vi "Launch.vi"(8 "error in (no error)":errorcluster, 10 "Mediator":refnum<class "IMediator.lvclass">, 11 "IMediatorBusMonitor (Type)":refnum<class "IMediatorBusMonitor.lvclass">) -> (0 "error out":errorcluster, 1 "Bus Monitor Enqueuer":refnum<class "Message Enqueuer.lvclass">, 2 "Mediator Out":refnum<class "IMediator.lvclass">, 3 "Notification Msg Type":refnum<class "Notification Msg.lvclass">)   [LabVIEW 2017, in "IMediator.lvlib" / "IMediatorBusMonitor.lvclass"]
uses:
  IMediatorBusMonitor.lvclass
  IMediator/IMediator.lvclass
  <vilib>/ActorFramework/Message Enqueuer/Message Enqueuer.lvclass
  gpm_packages/@cs/transport/Source/Concrete/ActorMessageTransport/Notification Msg/Notification Msg.lvclass
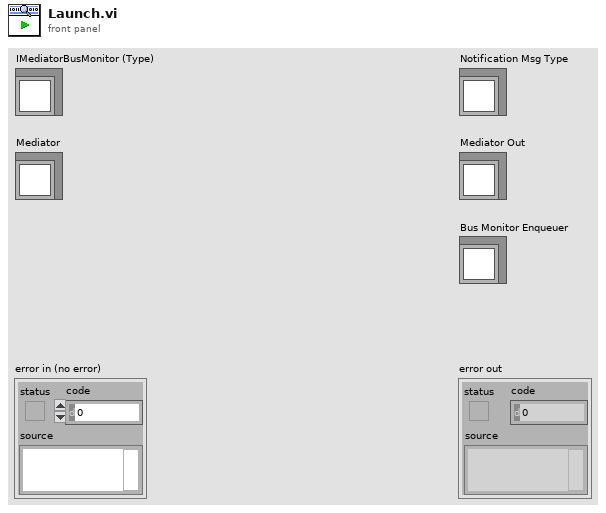
[diagram p1: front panel]
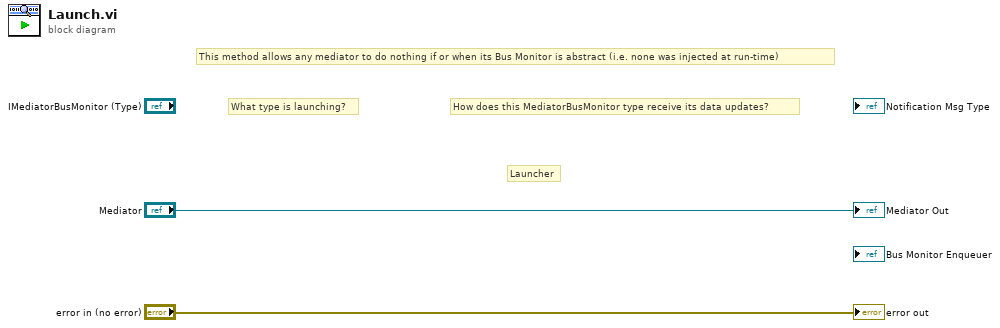
[diagram p0: block diagram]
diagram:
  # "Launcher"
  # "What type is launching?"
  # "How does this MediatorBusMonitor type receive its data updates?"
  # "This method allows any mediator to do nothing if or when its Bus Monitor is abstract (i.e. none was injected at run-time)"
  "error out" <- "error in (no error)"
  "Mediator Out" <- "Mediator"
